vi "Containers by Target.vi"(7 "Target Name":string, 10 "Targets":refnum<vi>[](array[refnum])) -> (1 "Container Names":string[](array[string]), 2 "Container Refs":refnum<vi>[](array[refnum]), 3 "Target":refnum<vi>)   [LabVIEW 2020, in "Conditum-Tools.lvlib" / "Entity Editor.lvclass"]
uses:
  Entity Editor.lvclass
  Entity Editor.lvclass/Entity Editor.ctl
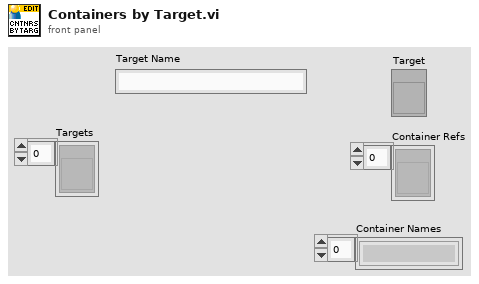
[diagram p1: front panel]
types:
  T1 = enum32{"invalid scope", "public", "private", "protected", "community"}
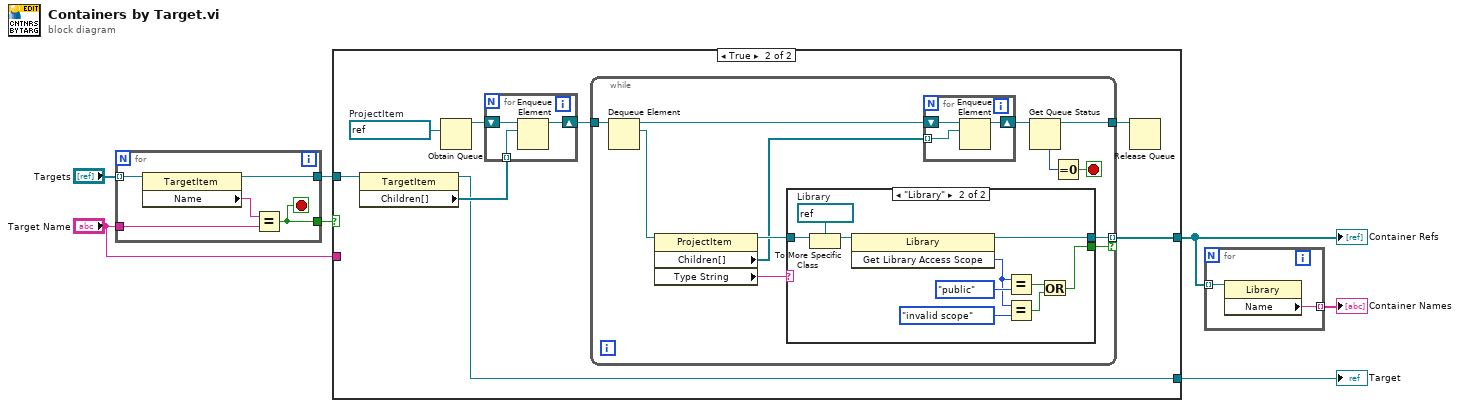
[diagram p0: block diagram]
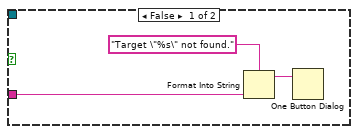
[diagram p2: hidden frame]
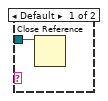
[diagram p3: hidden frame]
diagram:
  n1 = for {
    tunnel: "Targets" -> [w12] mode=indexing
    tunnel: "Target Name" -> [w11]
    tunnel: [w9] -> w5
    tunnel: [w8] -> w6
    stop <- w8 stop-if-true
    n2 = property class="TargetItem"(reference=w12) -> (reference out=w9:refnum<vi>, "Name"=w10:string)  [unwired: 1 in, 1 out]
    n3 = Equal?(x=w10, y=w11) -> (x = y?=w8:bool)
  }
  n4 = case shown="True" w6 {
    tunnel: w5 -> [_ w23]
    tunnel: [_ w17] -> w3
    tunnel: "Target Name" -> [w15 _]
    tunnel: [_ w16] -> w1
    frame False {
      n5 = Format Into String(format string="Target \"%s\" not found.", w15) -> (resulting string=w13:string)  [unwired: 2 in, 1 out]
      n6 = One Button Dialog(message=w13) -> ()  [unwired: 1 in, 1 out]
    }
    frame True {
      w22 = refnum<vi> refnum  # ProjectItem
      n7 = property class="TargetItem"(reference=w23) -> (reference out=w16:refnum<vi>, "Children[]"=w20:refnum<vi>[])  [unwired: 1 in, 1 out]
      n8 = Obtain Queue(element data type=w22) -> (queue out=w21:refnum<queue>)  [unwired: 4 in, 2 out]
      n9 = for {
        shift-right: [w50] -> w19
        shift-left: w21 -> [w52]
        tunnel: w20 -> [w51] mode=indexing
        n10 = Enqueue Element(queue=w52, element=w51) -> (queue out=w50:refnum<queue>)  [unwired: 2 in, 2 out]
      }
      n11 = while {
        tunnel: w19 -> [w35]
        tunnel: [w34] -> w18
        tunnel: [w26] -> w17 mode=indexing if=w25
        stop <- w32 stop-if-true
        n12 = Dequeue Element(queue=w35) -> (queue out=w31:refnum<queue>, element=w29:refnum<vi>)  [unwired: 2 in, 2 out]
        n13 = property class="ProjectItem"(reference=w29) -> (reference out=w27:refnum<vi>, "Children[]"=w24:refnum<vi>[], "Type String"=w28:string)  [unwired: 1 in, 1 out]
        n14 = case shown="\"Library\"" w28 {
          tunnel: w27 -> [w36 w46]
          tunnel: [_ w39] -> w26
          tunnel: [_ w37] -> w25
          frame Default {
            n15 = Close Reference(reference=w36) -> ()  [unwired: 1 in, 1 out]
          }
          frame "Library" {
            w45 = refnum<vi> refnum  # Library
            n16 = To More Specific Class(target class=w45, reference=w46) -> (specific class reference=w38:refnum<vi>)  [unwired: 1 in, 1 out]
            n17 = invoke class="Library" method="Get Library Access Scope"(reference=w38) -> (reference out=w39:refnum<vi>, "Get Library Access Scope"=w42:T1)  [unwired: 2 in, 1 out]
            n18 = Equal?(x=w42, y=T1."public") -> (x = y?=w41:bool)
            n19 = Equal?(x=w42, y=T1."invalid scope") -> (x = y?=w40:bool)
            n20 = Or(x=w41, y=w40) -> (x .or. y?=w37:bool)
          }
        }
        n21 = for {
          shift-right: [w48] -> w30
          shift-left: w31 -> [w49]
          tunnel: w24 -> [w47] mode=indexing
          n22 = Enqueue Element(queue=w49, element=w47) -> (queue out=w48:refnum<queue>)  [unwired: 2 in, 2 out]
        }
        n23 = Get Queue Status(queue=w30) -> (queue out=w34:refnum<queue>, # elements in queue=w33:i32)  [unwired: 2 in, 6 out]
        n24 = Equal To 0?(x=w33) -> (x = 0?=w32:bool)
      }
      n25 = Release Queue(queue=w18) -> ()  [unwired: 2 in, 3 out]
    }
  }
  "Container Refs" <- w3
  "Target" <- w1
  n26 = for {
    tunnel: w3 -> [w54] mode=indexing
    tunnel: [w53] -> w2 mode=indexing
    n27 = property class="Library"(reference=w54) -> ("Name"=w53:string)  [unwired: 1 in, 2 out]
  }
  "Container Names" <- w2
